vi "Pulse Parameters.vi"(0 "X":dbl[](array[numeric])) -> (2 "slew rate":dbl format="%0.2f", 3 "overshoot":dbl format="%0.2f", 4 "risetime":dbl format="%0.2f", 6 "top":dbl format="%0.2f", 8 "amplitude":dbl format="%0.2f", 10 "base":dbl format="%0.2f", 11 "delay":dbl format="%0.2f", 12 "duration":dbl format="%0.2f", 13 "falltime":dbl format="%0.2f", 14 "error":i32, 15 "undershoot":dbl format="%0.2f")   [LabVIEW 2018, in "NI_AALPro.lvlib"]
doc: "Analyzes the input sequence <B>X</B> for a pulse pattern and determines the best set of pulse parameters that describes the pulse."
uses:
  <vilib>/Analysis/NI_AALPro.lvlib
  <resource>/lvanlys.dll
panel:
  # "Pulse Parameters"
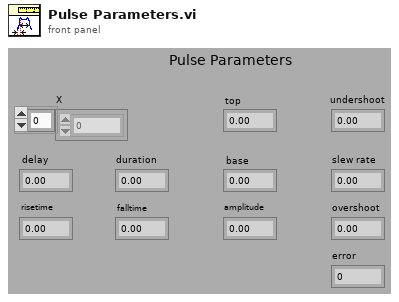
[diagram p1: front panel]
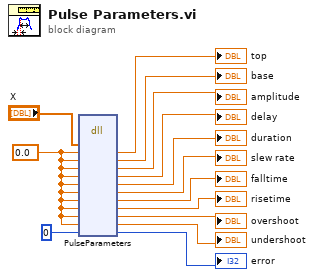
[diagram p0: block diagram]
diagram:
  w13 = 0.0 ("top")
  n1 = dll-call lib="C:/Program Files (x86)/National Instruments/LabVIEW 2018/resource/lvanlys.*" fn="PulseParameters"("X"="X", "top"=w13, "base"=w13, "amplitude"=w13, "delay"=w13, "width"=w13, "slew rate"=w13, "falltime"=w13, "risetime"=w13, "overshoot"=w13, "undershoot"=w13, "error"=0) -> ("top"=→"top":dbl, "base"=→"base":dbl, "amplitude"=→"amplitude":dbl, "delay"=→"delay":dbl, "width"=→"duration":dbl, "slew rate"=→"slew rate":dbl, "falltime"=→"falltime":dbl, "risetime"=→"risetime":dbl, "overshoot"=→"overshoot":dbl, "undershoot"=→"undershoot":dbl, "error"=→"error":i32)  [unwired: 5 in, 2 out]
